vi "Get Task.vi"(8 "error in (no error)":errorcluster, 10 "Task Name":string, 11 "Series Base in":refnum<class "Series Base.lvclass">) -> (0 "error out":errorcluster, 2 "Task":refnum<class "Task Base.lvclass">, 3 "Series Base out":refnum<class "Series Base.lvclass">)   [LabVIEW 2023, in "HAL GOOP4.lvlib" / "Series Base.lvclass"]
uses:
  Series Base.lvclass
  Task/Task Base/Task Base.lvclass
  Series Base.lvclass/Series Base.ctl
  <vilib>/Utility/error.llb/Error Cluster From Error Code.vi
  <vilib>/ErrorRing/Error Ring.xnode
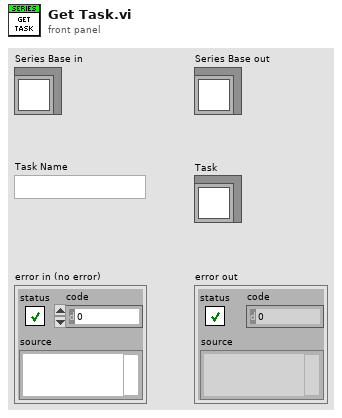
[diagram p1: front panel]
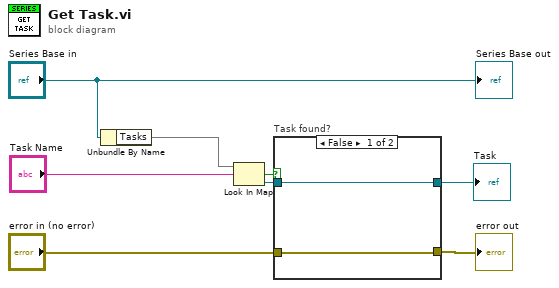
[diagram p0: block diagram]
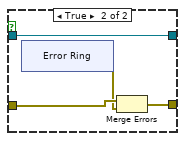
[diagram p2: hidden frame]
diagram:
  n1 = Unbundle By Name("Series Base in") -> ("Tasks"=w3:map{string, refnum<class "Task Base.lvclass">})
  n2 = Look In Map(map=w3, key="Task Name") -> (key not found?=w2:bool, value=w1:refnum<class "Task Base.lvclass">)  [unwired: 1 in]
  n3 = case "Task found?" shown="False" w2 {
    tunnel: w1 -> [w10 w14]
    tunnel: [w10 w14] -> w4
    tunnel: "error in (no error)" -> [w9 w13]
    tunnel: [w9 w11] -> w7
    frame False {
    }
    frame True {
      n4 = xnode "Error Ring"() -> ("error out"=w12:errorcluster)
      n5 = Merge Errors(w13, w12) -> (w11:errorcluster)
    }
  }
  "error out" <- w7
  "Task" <- w4
  "Series Base out" <- "Series Base in"
